vi "Last Ack Creator Queue.vi"(10 "Queue":refnum<class "Queue.lvclass">, 11 "Template Queue in":refnum<class "Template Queue.lvclass">) -> (3 "Template Queue out":refnum<class "Template Queue.lvclass">)   [LabVIEW 2021, in "_Template.lvlib" / "Templates.lvlib" / "Template Queue.lvlib" / "Template Queue.lvclass"]
uses:
  Template Queue.lvclass
  <vilib>/jettl/jettl/jettl/Queue/Queue.lvclass
  Template Queue.lvclass/Template Queue.ctl
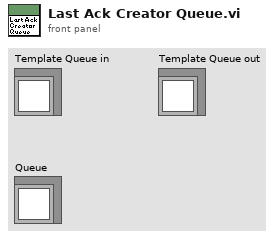
[diagram p1: front panel]
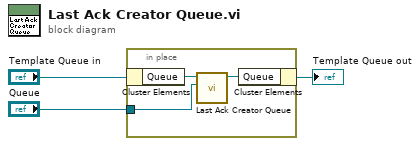
[diagram p0: block diagram]
diagram:
  n1 = in-place {
    in-place-border: "Queue" -> [w4]
    n2 = in-place-cluster #1("Template Queue in") -> ("Queue"=w6:refnum<class "Queue.lvclass">)
    n3 = call-dynamic "Last Ack Creator Queue.vi"("Queue"=w4, "jettl Msg Last Ack Creator Queue in"=w6) -> ("jettl Msg Last Ack Creator Queue out"=w5:refnum<class "Queue.lvclass">)  [unwired: 9 in]
    n4 = in-place-cluster #1("Queue"=w5) -> (→"Template Queue out":refnum<class "Template Queue.lvclass">)
  }
